vi "FdxInitTxFrameHeaderCvi.vi"(8 "error in":errorcluster) -> (0 "error out":errorcluster, 1 "TxFrameHeader":T1)   [LabVIEW 2020, in "AIM664LV.lvlib"]
doc: "This function initializes a Transmit Frame Header Structure for Standard Frame (No Instruction Type). This structure is used for defining a Generic Transmit Queue entry with the AiFdxCmdTxQueueWrite function."
uses:
  AIM664LV.lvlib
  AFDX_LibraryAdmin/FdxGlobalDllPath.vi
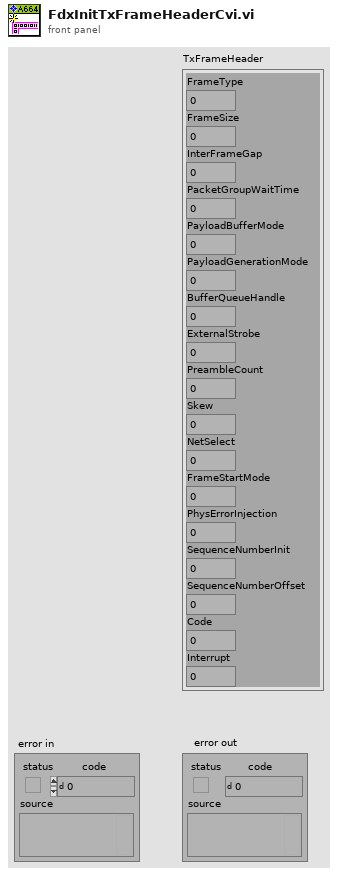
[diagram p1: front panel]
types:
  T1 = cluster{"FrameType":u8, "FrameSize":u16, "InterFrameGap":u32, "PacketGroupWaitTime":u32, "PayloadBufferMode":u8, "PayloadGenerationMode":u8, "BufferQueueHandle":u32, "ExternalStrobe":u8, "PreambleCount":u8, "Skew":u32, "NetSelect":u8, "FrameStartMode":u8, "PhysErrorInjection":u32, "SequenceNumberInit":u16, "SequenceNumberOffset":u16, "Code":u8, "Interrupt":u8}
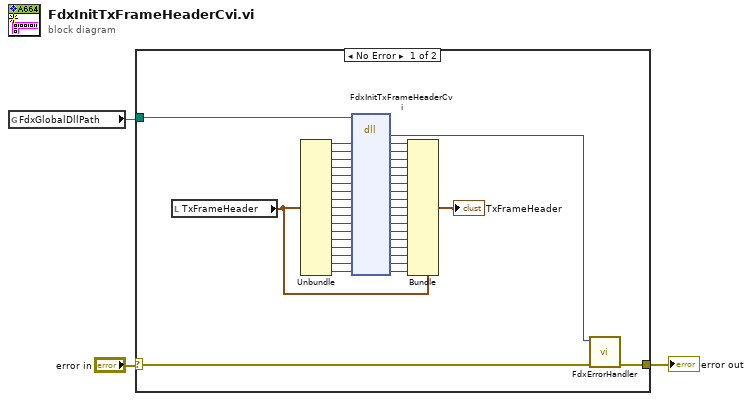
[diagram p0: block diagram]
diagram:
  n1 = global read "FdxGlobalDllPath.vi" "FdxGlobalDllPath"() -> (w1:path)
  n2 = case shown="No Error" "error in" {
    selector: "error in" -> [w42 w44]
    tunnel: [w43 w44] -> w3
    tunnel: w1 -> [w4 _]
    frame No Error {
      n3 = local read "TxFrameHeader"() -> (w30:T1)
      n4 = Unbundle(w30) -> ("FrameType"=w21:u8, "FrameSize"=w20:u16, "InterFrameGap"=w19:u32, "PacketGroupWaitTime"=w18:u32, "PayloadBufferMode"=w17:u8, "PayloadGenerationMode"=w16:u8, "BufferQueueHandle"=w15:u32, "ExternalStrobe"=w14:u8, "PreambleCount"=w13:u8, "Skew"=w12:u32, "NetSelect"=w11:u8, "FrameStartMode"=w10:u8, "PhysErrorInjection"=w9:u32, "SequenceNumberInit"=w8:u16, "SequenceNumberOffset"=w7:u16, "Code"=w6:u8, "Interrupt"=w5:u8)
      n5 = dll-call lib="aim_fdx.19.dll" fn="FdxInitTxFrameHeaderCvi"(path in=w4, "FrameType"=w21, "FrameSize"=w20, "InterFrameGap"=w19, "PacketGroupWaitTime"=w18, "PayloadBufferMode"=w17, "PayloadGenerationMode"=w16, "BufferQueueHandle"=w15, "ExternalStrobe"=w14, "PreambleCount"=w13, "Skew"=w12, "NetSelect"=w11, "FrameStartMode"=w10, "PhysErrorInjection"=w9, "SequenceNumberInit"=w8, "SequenceNumberOffset"=w7, "Code"=w6, "Interrupt"=w5) -> ("status"=w41:i32, "FrameType"=w39:u8, "FrameSize"=w38:u16, "InterFrameGap"=w37:u32, "PacketGroupWaitTime"=w36:u32, "PayloadBufferMode"=w35:u8, "PayloadGenerationMode"=w34:u8, "BufferQueueHandle"=w33:u32, "ExternalStrobe"=w32:u8, "PreambleCount"=w31:u8, "Skew"=w29:u32, "NetSelect"=w28:u8, "FrameStartMode"=w27:u8, "PhysErrorInjection"=w26:u32, "SequenceNumberInit"=w25:u16, "SequenceNumberOffset"=w24:u16, "Code"=w23:u8, "Interrupt"=w22:u8)  [unwired: 2 in, 2 out]
      n6 = Bundle(cluster=w30, "FrameType"=w39, "FrameSize"=w38, "InterFrameGap"=w37, "PacketGroupWaitTime"=w36, "PayloadBufferMode"=w35, "PayloadGenerationMode"=w34, "BufferQueueHandle"=w33, "ExternalStrobe"=w32, "PreambleCount"=w31, "Skew"=w29, "NetSelect"=w28, "FrameStartMode"=w27, "PhysErrorInjection"=w26, "SequenceNumberInit"=w25, "SequenceNumberOffset"=w24, "Code"=w23, "Interrupt"=w22) -> (→"TxFrameHeader":T1)
      n7 = call "FdxErrorHandler.vi"("error in"=w42, "AIM Error"=w41) -> ("error out"=w43:errorcluster)  [unwired: 9 in]
    }
    frame Error {
    }
  }
  "error out" <- w3
